vi "Get Output Uncertainty.vi"(8 "error in (no error)":errorcluster, 9 "Specified Uncertainty (0: 90-days)":u32(ring) items=["90-days", "365-days"], 10 "Output (T: Primary)":bool=TRUE, 11 "VISA resource name":refnum<visa-resource-name>) -> (0 "error out":errorcluster, 1 "Output Uncertainty Units":i32, 2 "Output Uncertainty":dbl format="%.4f", 3 "VISA resource name out":refnum<visa-resource-name>, 4 "Specification Interval":i32)   [LabVIEW 2014, in "Fluke 5XXX Series Multicalibrators.lvlib"]
doc: "This VI returns specified uncertainties for the present output. If there are no specifications for an output, returns value less or equal to zero."
uses:
  Fluke 5XXX Series Multicalibrators.lvlib
panel:
  # "Primary"
  # "Secondary"
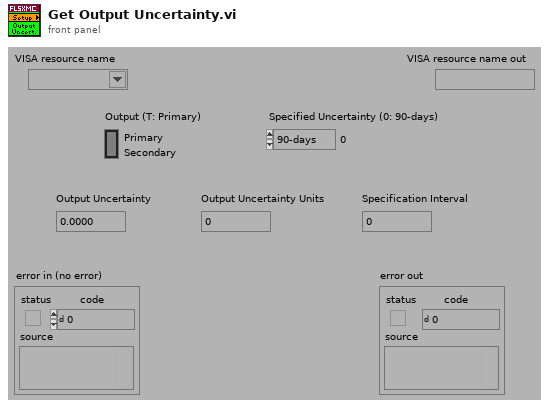
[diagram p1: front panel]
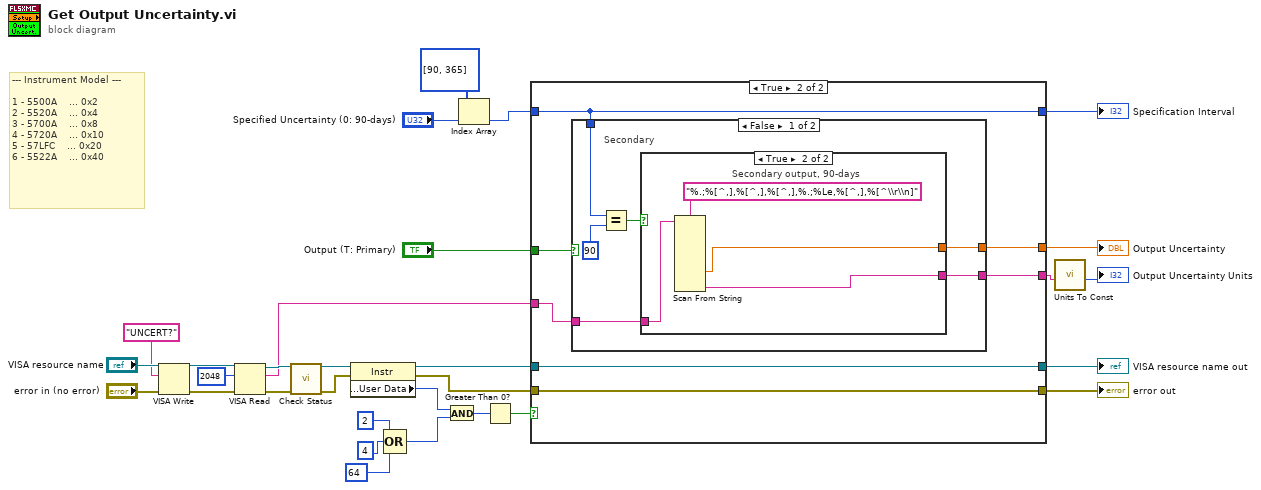
[diagram p0: block diagram]
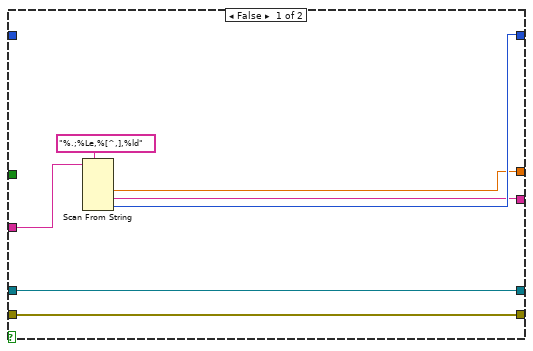
[diagram p2: hidden frame]
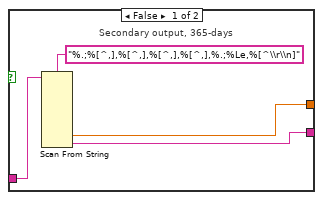
[diagram p3: hidden frame]
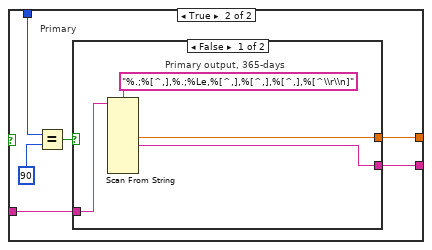
[diagram p4: hidden frame]
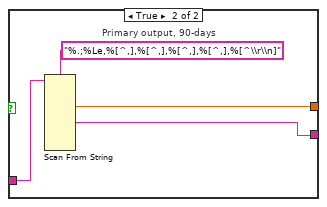
[diagram p5: hidden frame]
diagram:
  # "--- Instrument Model ---\n\n1 - 5500A    ... 0x2\n2 - 5520A    ... 0x4\n3 - 5700A    ... 0x8\n4 - 5720A    ... 0x10\n5 - 57LFC    ... 0x20\n6 - 5522A    ... 0x40"
  n1 = VISA Write(VISA resource name="VISA resource name", write buffer="UNCERT?", error in (no error)="error in (no error)") -> (VISA resource name out=w18:refnum<visa-resource-name>, error out=w17:errorcluster)  [unwired: 1 out]
  n2 = VISA Read(VISA resource name=w18, byte count=u32 2048 ("byte count (0)"), error in (no error)=w17) -> (VISA resource name out=w14:refnum<visa-resource-name>, read buffer=w11:string, error out=w15:errorcluster)  [unwired: 1 out]
  n3 = call "Check Status.vi"("VISA resource name"=w14, "error in (no error)"=w15) -> ("VISA resource name out"=w9:refnum<visa-resource-name>, "error out"=w7:errorcluster)  [unwired: 12 in]
  n4 = property class="Instr"(reference=w9, error in=w7) -> (reference out=w8:refnum<visa-resource-name>, error out=w6:errorcluster, "General Settings:User Data"=w5:u32)
  n5 = Compound Arithmetic op=OR(u32 2 ("Numeric"), u32 4 ("Numeric"), 64 ("Numeric")) -> (w4:u32)
  n6 = And(x=w5, y=w4) -> (x .and. y?=w3:u32)
  n7 = Index Array(array=i32[] [90, 365] ("Specified Uncertainty arr"), index="Specified Uncertainty (0: 90-days)") -> (element=w28:i32)
  n8 = Greater Than 0?(x=w3) -> (x > 0?=w2:bool)
  n9 = case shown="True" w2 {
    tunnel: w28 -> [_ w42]
    tunnel: [w35 w42] -> w27
    tunnel: "Output (T: Primary)" -> [_ w44]
    tunnel: w11 -> [w36 w43]
    tunnel: w8 -> [w32 w38]
    tunnel: [w33 w41] -> w25
    tunnel: [w34 w40] -> w10
    tunnel: [w32 w38] -> w22
    tunnel: w6 -> [w31 w39]
    tunnel: [w31 w39] -> w23
    frame False {
      n10 = Scan From String(format string="%.;%Le,%[^,],%ld", input string=w36) -> (output 1=w33:dbl, output 2=w34:string, output 3=w35:i32)  [unwired: 5 in, 3 out]
    }
    frame True {
      n11 = case shown="False" w44 {
        tunnel: w43 -> [w48 w64]
        tunnel: w42 -> [w47 w61]
        tunnel: [w46 w60] -> w41
        tunnel: [w45 w59] -> w40
        frame False {
          # "Secondary"
          n12 = Equal?(x=w47, y=90) -> (x = y?=w50:bool)
          n13 = case shown="True" w50 {
            tunnel: w48 -> [w53 w57]
            tunnel: [w52 w56] -> w46
            tunnel: [w51 w55] -> w45
            frame False {
              # "Secondary output, 365-days"
              n14 = Scan From String(format string="%.;%[^,],%[^,],%[^,],%[^,],%.;%Le,%[^\\r\\n]", input string=w53) -> (output 5=w52:dbl, output 6=w51:string)  [unwired: 12 in, 3 out]
            }
            frame True {
              # "Secondary output, 90-days"
              n15 = Scan From String(format string="%.;%[^,],%[^,],%[^,],%.;%Le,%[^,],%[^\\r\\n]", input string=w57) -> (output 4=w56:dbl, output 6=w55:string)  [unwired: 12 in, 3 out]
            }
          }
        }
        frame True {
          # "Primary"
          n16 = Equal?(x=w61, y=90) -> (x = y?=w63:bool)
          n17 = case shown="False" w63 {
            tunnel: w64 -> [w67 w71]
            tunnel: [w66 w70] -> w60
            tunnel: [w65 w69] -> w59
            frame False {
              # "Primary output, 365-days"
              n18 = Scan From String(format string="%.;%[^,],%.;%Le,%[^,],%[^,],%[^,],%[^\\r\\n]", input string=w67) -> (output 2=w66:dbl, output 3=w65:string)  [unwired: 12 in, 3 out]
            }
            frame True {
              # "Primary output, 90-days"
              n19 = Scan From String(format string="%.;%Le,%[^,],%[^,],%[^,],%[^,],%[^\\r\\n]", input string=w71) -> (output 1=w70:dbl, output 3=w69:string)  [unwired: 12 in, 3 out]
            }
          }
        }
      }
    }
  }
  "Output Uncertainty" <- w25
  "Specification Interval" <- w27
  "VISA resource name out" <- w22
  "error out" <- w23
  n20 = call "Units To Const.vi"("Units"=w10) -> ("Const"=→"Output Uncertainty Units":i32)  [unwired: 10 in]
